vi "WriteMoxa8.vi"(0 "PORT LAUDA 1":dbl, 1 "DATA LAUDA 1":dbl, 2 "enable2":i32, 4 "DATA ISMA 1":dbl, 6 "DATA ISMA 2":dbl, 7 "enable1":i32, 9 "PORT ISMA 1":dbl, 10 "DATA ISMA 3":dbl, 11 "PORT ISMA 2":dbl, 12 "PORT ISMA 3":dbl, 14 "enable3":i32) -> ()   [LabVIEW 2017]
uses:
  BERTTA.dll
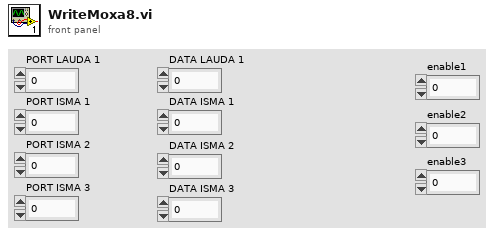
[diagram p1: front panel]
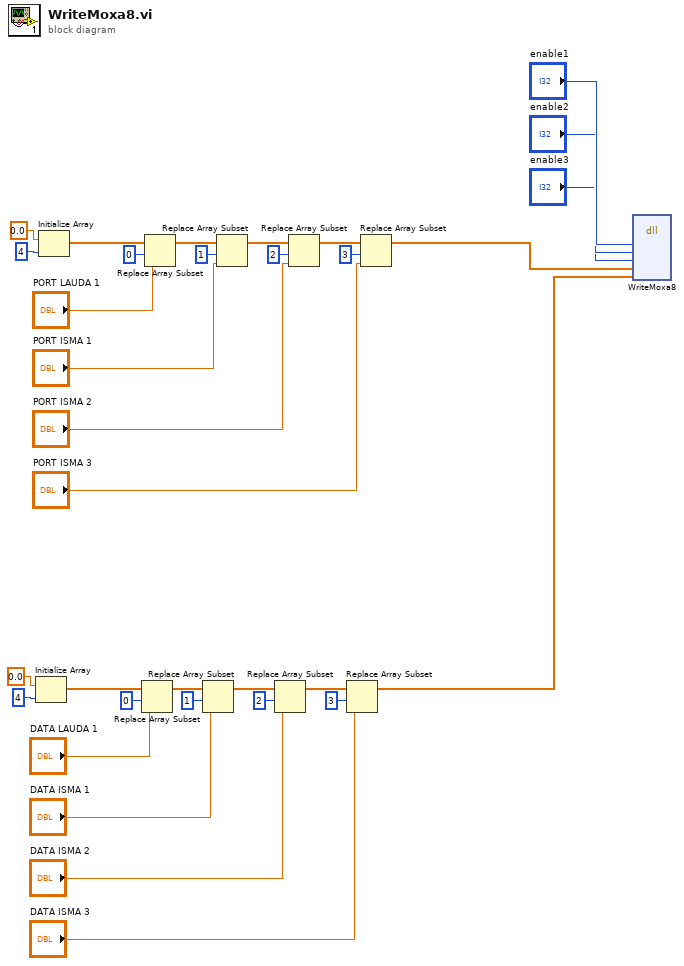
[diagram p0: block diagram]
diagram:
  n1 = Initialize Array(0.0 ("element"), 4 ("dimension size")) -> (w20:dbl[])
  n2 = Initialize Array(0.0 ("element"), 4 ("dimension size")) -> (w31:dbl[])
  n3 = Replace Array Subset(array=w20, new element="DATA LAUDA 1", index=0) -> (w1:dbl[])
  n4 = Replace Array Subset(array=w31, new element="PORT LAUDA 1", index=0) -> (w30:dbl[])
  n5 = Replace Array Subset(array=w1, new element="DATA ISMA 1", index=1) -> (w19:dbl[])
  n6 = Replace Array Subset(array=w30, new element="PORT ISMA 1", index=1) -> (w29:dbl[])
  n7 = Replace Array Subset(array=w19, new element="DATA ISMA 2", index=2) -> (w18:dbl[])
  n8 = Replace Array Subset(array=w29, new element="PORT ISMA 2", index=2) -> (w28:dbl[])
  n9 = Replace Array Subset(array=w18, new element="DATA ISMA 3", index=3) -> (w2:dbl[])
  n10 = Replace Array Subset(array=w28, new element="PORT ISMA 3", index=3) -> (w3:dbl[])
  n11 = dll-call lib="C:/Users/shresplab/OneDrive - Kemira Oyj/Documents/GitHub/Bertta/BERTTA/x64/Debug/BERTTA.dll" fn="WriteMoxa8"("enable1"="enable1", "enable2"="enable2", "enable3"="enable3", "ports"=w3, "params"=w2) -> ()  [unwired: 9 in, 2 out]
